vi "navX GetSetRefnum.vi"(8 "error in (no error)":errorcluster, 9 "menu":enum16{"set", "get", "delete"}(ring), 10 "refnum name":string, 11 "navX Device TypeDef":T1={"navX Interface Protocol"=enum."SPI", "navX Interface Protocol TypeDefs"={"SPIDevRef"={"DevStatus"={"status"=FALSE, "code"=0, "source"=""}, "Handle"=0, "SPI Bus"=enum."SPI On-Board, CS0"}, "I2CDevRef"={"DevStatus"={"status"=FALSE, "code"=0, "source"=""}, "Device Address"=0, "Handle"=0, "I2C Bus"=enum."Invalid"}}, "navX System Information"={"Board Information"={"WhoAmI (50 | 0x32)"=0, "Board Revision"=0, "Firmware Major Version"=0, "Firmware Minor Version"=0}, "Status"={"Update Rate Hz"=0, "Accelerometer Full-Scale Range"=0, "Gyro Full-Scale Range"=0, "NAVX_OP_STATUS"=0, "NAVX_CAL_STATUS"=0, "NAVX_SELFTEST_STATUS"=0, "NAVX_SENSOR_STATUS"={"MOVING"=FALSE, "YAW_STABLE"=FALSE, "MAG_DISTURBANCE"=FALSE, "ALTITUDE_VALID"=FALSE, "SEALEVEL_PRESS_SET"=FALSE, "FUSED_HEADING_VALID"=FALSE}}, "Offsets"={"Yaw"=0.0, "Quat W"=0.0, "Quat X"=0.0, "Quat Y"=0.0, "Quat Z"=0.0}}, "navX Common Information"={"Update Rate (4Hz-60Hz)"=50, "refnum name"="", "error"={"status"=FALSE, "code"=0, "source"=""}}} {"navX Common Information"."Update Rate (4Hz-60Hz)" min=4 max=50 step=1; "navX System Information"."Status"."NAVX_OP_STATUS" items=["INITIALIZING", "SELFTEST_IN_PROGRESS", "ERROR", "IMU_AUTOCAL_IN_PROGRESS", "NORMAL"]; "navX System Information"."Status"."NAVX_CAL_STATUS" items=["IMU_CAL_STATE_MASK"=3, "IMU_CAL_INPROGRESS"=0, "IMU_CAL_ACCUMULATE"=1, "IMU_CAL_COMPLETE"=2, "MAG_CAL_COMPLETE"=4, "BARO_CAL_COMPLETE"=8]; "navX Interface Protocol TypeDefs"."I2CDevRef"."Device Address" format="%.0x"}) -> (0 "error out":errorcluster, 3 "navX Device TypeDef":T1={"navX Interface Protocol"=enum."SPI", "navX Interface Protocol TypeDefs"={"SPIDevRef"={"DevStatus"={"status"=FALSE, "code"=0, "source"=""}, "Handle"=0, "SPI Bus"=enum."SPI On-Board, CS0"}, "I2CDevRef"={"DevStatus"={"status"=FALSE, "code"=0, "source"=""}, "Device Address"=0, "Handle"=0, "I2C Bus"=enum."Invalid"}}, "navX System Information"={"Board Information"={"WhoAmI (50 | 0x32)"=0, "Board Revision"=0, "Firmware Major Version"=0, "Firmware Minor Version"=0}, "Status"={"Update Rate Hz"=0, "Accelerometer Full-Scale Range"=0, "Gyro Full-Scale Range"=0, "NAVX_OP_STATUS"=0, "NAVX_CAL_STATUS"=0, "NAVX_SELFTEST_STATUS"=0, "NAVX_SENSOR_STATUS"={"MOVING"=FALSE, "YAW_STABLE"=FALSE, "MAG_DISTURBANCE"=FALSE, "ALTITUDE_VALID"=FALSE, "SEALEVEL_PRESS_SET"=FALSE, "FUSED_HEADING_VALID"=FALSE}}, "Offsets"={"Yaw"=0.0, "Quat W"=0.0, "Quat X"=0.0, "Quat Y"=0.0, "Quat Z"=0.0}}, "navX Common Information"={"Update Rate (4Hz-60Hz)"=50, "refnum name"="", "error"={"status"=FALSE, "code"=0, "source"=""}}} {"navX Common Information"."Update Rate (4Hz-60Hz)" min=4 max=50 step=1; "navX System Information"."Status"."NAVX_OP_STATUS" items=["INITIALIZING", "SELFTEST_IN_PROGRESS", "ERROR", "IMU_AUTOCAL_IN_PROGRESS", "NORMAL"]; "navX System Information"."Status"."NAVX_CAL_STATUS" items=["IMU_CAL_STATE_MASK"=3, "IMU_CAL_INPROGRESS"=0, "IMU_CAL_ACCUMULATE"=1, "IMU_CAL_COMPLETE"=2, "MAG_CAL_COMPLETE"=4, "BARO_CAL_COMPLETE"=8]; "navX Interface Protocol TypeDefs"."I2CDevRef"."Device Address" format="%.0x"})   [LabVIEW 2015, in "navX-MXP IMU.lvlib"]
uses:
  navX-MXP IMU.lvlib
  TypeDefs/navX Device TypeDef.ctl
  TypeDefs/Value TypeDefs/navX Interface Protocol.ctl
  <vilib>/Rock Robotics/WPI/SPI/WPI_SPIDevRef.ctl
  <vilib>/Rock Robotics/SystemInterfaces/spilib/spi_bus.ctl
  <vilib>/Rock Robotics/WPI/I2C/WPI_I2CDevRef.ctl
  <vilib>/Rock Robotics/SystemInterfaces/i2clib/i2c_bus.ctl
  TypeDefs/Data TypeDefs/navX Board Information.ctl
  TypeDefs/Data TypeDefs/navX Status Data.ctl
  TypeDefs/Value TypeDefs/navX NAVX_OP_STATUS.ctl
  TypeDefs/Value TypeDefs/navX NAVX_CAL_STATUS.ctl
  TypeDefs/Value TypeDefs/navX NAVX_SENSOR_STATUS.ctl
  TypeDefs/Data TypeDefs/navX Offsets Data.ctl
  TypeDefs/Value TypeDefs/navX Update Rate.ctl
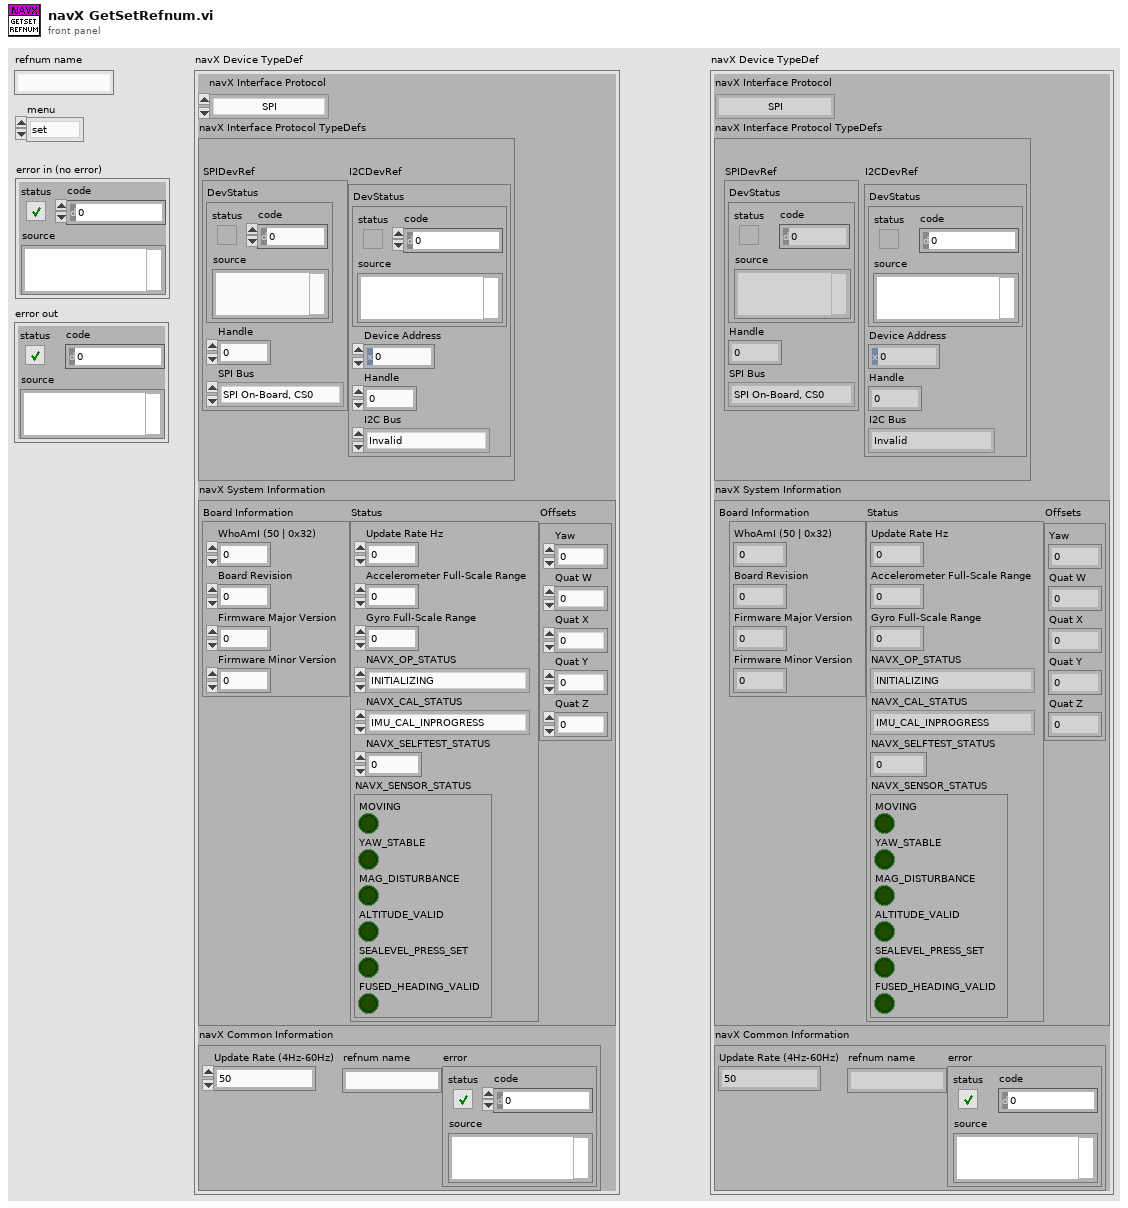
[diagram p1: front panel]
types:
  T1 = typedef "navX-MXP IMU.lvlib/navX Device TypeDef.ctl" = cluster{"navX Interface Protocol":T2, "navX Interface Protocol TypeDefs":cluster{"SPIDevRef":T3, "I2CDevRef":T5}, "navX System Information":cluster{"Board Information":T7, "Status":T8, "Offsets":T12}, "navX Common Information":cluster{"Update Rate (4Hz-60Hz)":T13, "refnum name":string, "error":errorcluster}}
  T2 = typedef "navX-MXP IMU.lvlib/navX Interface Protocol.ctl" = enum16{"SPI", "I2C"}
  T3 = typedef "WPI_SPIDevRef.ctl" = cluster{"DevStatus":errorcluster, "Handle":i32, "SPI Bus":T4}
  T4 = typedef "spi_bus.ctl" = enum16{"SPI On-Board, CS0", "SPI On-Board, CS1", "SPI On-Board, CS2", "SPI On-Board, CS3", "SPI MXP", "Invalid"}
  T5 = typedef "WPI_I2CDevRef.ctl" = cluster{"DevStatus":errorcluster, "Device Address":u8, "Handle":i32, "I2C Bus":T6}
  T6 = typedef "i2c_bus.ctl" = enum16{"I2C On-Board", "I2C MXP", "Invalid"}
  T7 = typedef "navX-MXP IMU.lvlib/navX Board Information.ctl" = cluster{"WhoAmI (50 | 0x32)":u8, "Board Revision":u8, "Firmware Major Version":u8, "Firmware Minor Version":u8}
  T8 = typedef "navX-MXP IMU.lvlib/navX Status Data.ctl" = cluster{"Update Rate Hz":u8, "Accelerometer Full-Scale Range":u8, "Gyro Full-Scale Range":u16, "NAVX_OP_STATUS":T9, "NAVX_CAL_STATUS":T10, "NAVX_SELFTEST_STATUS":u8, "NAVX_SENSOR_STATUS":T11}
  T9 = typedef "navX-MXP IMU.lvlib/navX NAVX_OP_STATUS.ctl" = u8
  T10 = typedef "navX-MXP IMU.lvlib/navX NAVX_CAL_STATUS.ctl" = u8
  T11 = typedef "navX-MXP IMU.lvlib/navX NAVX_SENSOR_STATUS.ctl" = cluster{"MOVING":bool, "YAW_STABLE":bool, "MAG_DISTURBANCE":bool, "ALTITUDE_VALID":bool, "SEALEVEL_PRESS_SET":bool, "FUSED_HEADING_VALID":bool}
  T12 = typedef "navX-MXP IMU.lvlib/navX Offsets Data.ctl" = cluster{"Yaw":dbl, "Quat W":dbl, "Quat X":dbl, "Quat Y":dbl, "Quat Z":dbl}
  T13 = typedef "navX-MXP IMU.lvlib/navX Update Rate.ctl" = u8
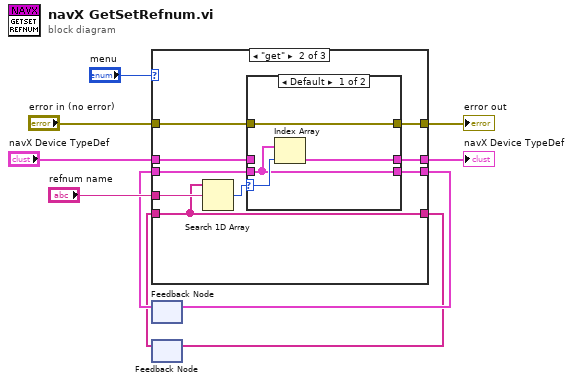
[diagram p0: block diagram]
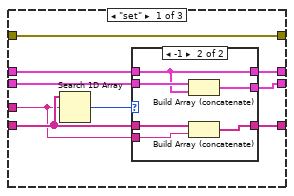
[diagram p2: hidden frame]
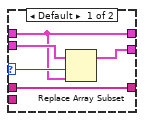
[diagram p3: hidden frame]
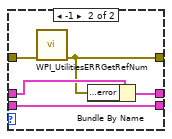
[diagram p4: hidden frame]
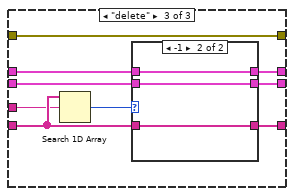
[diagram p5: hidden frame]
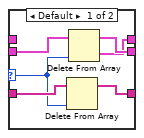
[diagram p6: hidden frame]
diagram:
  n1 = feedback #1() -> (w3:T1[])  [unwired: 1 in]
  n2 = feedback #2() -> (w1:string[])  [unwired: 1 in]
  n3 = case shown="\"get\"" "menu" {
    tunnel: "navX Device TypeDef" -> [w14 w36 w52]
    tunnel: [w13 w35 w51] -> w4
    tunnel: w3 -> [w15 w37 w53]
    tunnel: [w12 w34 w50] -> w6
    tunnel: [w19 w33 w57] -> w2
    tunnel: w1 -> [w18 w33 w56]
    tunnel: "refnum name" -> [w16 w38 w54]
    tunnel: [w11 w31 w49] -> w8
    tunnel: "error in (no error)" -> [w11 w32 w49]
    frame "set" {
      n4 = Search 1D Array(1D array=w18, element=w16) -> (index of element=w17:i32)  [unwired: 1 out]
      n5 = case shown="-1" w17 {
        selector: w17 -> [w22 _]
        tunnel: [w24 w30] -> w19
        tunnel: w18 -> [w24 w29]
        tunnel: w16 -> [_ w28]
        tunnel: w15 -> [w23 w27]
        tunnel: w14 -> [w20 w25]
        tunnel: [w21 w26] -> w13
        tunnel: [w20 w25] -> w12
        frame Default {
          n6 = Replace Array Subset(array=w23, new element=w20, index=w22) -> (w21:T1[])
        }
        frame -1 {
          n7 = Build Array (concatenate)(w27, w25) -> (w26:T1[])
          n8 = Build Array (concatenate)(w29, w28) -> (w30:string[])
        }
      }
    }
    frame "get" {
      n9 = Search 1D Array(1D array=w33, element=w38) -> (index of element=w39:i32)  [unwired: 1 out]
      n10 = case shown="Default" w39 {
        selector: w39 -> [w43 _]
        tunnel: w37 -> [w41 w48]
        tunnel: w36 -> [_ w46]
        tunnel: [w41 w48] -> w35
        tunnel: [w42 w45] -> w34
        tunnel: w32 -> [w40 w47]
        tunnel: [w40 w44] -> w31
        frame Default {
          n11 = Index Array(array=w41, index=w43) -> (element=w42:T1)
        }
        frame -1 {
          n12 = call <vilib>:"WPI_UtilitiesERRGetRefNum.vi"("error in (no error)"=w47) -> ("ERRGetRefNum"=w44:errorcluster)  [unwired: 10 out]
          n13 = Bundle By Name(cluster=w46, "navX Common Information.error"=w44) -> (w45:T1)
        }
      }
    }
    frame "delete" {
      n14 = Search 1D Array(1D array=w56, element=w54) -> (index of element=w55:i32)  [unwired: 1 out]
      n15 = case shown="-1" w55 {
        selector: w55 -> [w58 _]
        tunnel: [w59 w65] -> w57
        tunnel: w56 -> [w60 w65]
        tunnel: w53 -> [w63 w64]
        tunnel: w52 -> [_ w66]
        tunnel: [w62 w64] -> w51
        tunnel: [w61 w66] -> w50
        frame Default {
          n16 = Delete From Array(array=w60, index=w58) -> (array with subset deleted=w59:string[])  [unwired: 1 in, 1 out]
          n17 = Delete From Array(array=w63, index=w58) -> (deleted portion=w61:T1, array with subset deleted=w62:T1[])  [unwired: 1 in]
        }
        frame -1 {
        }
      }
    }
  }
  "error out" <- w8
  "navX Device TypeDef" <- w6
  n18 = feedback-in #1(w4) -> ()
  n19 = feedback-in #2(w2) -> ()
